vi "File.Remove Double Backslash from Path.vi"(11 "Path":path) -> (3 "Path Out":path)   [LabVIEW 2018]
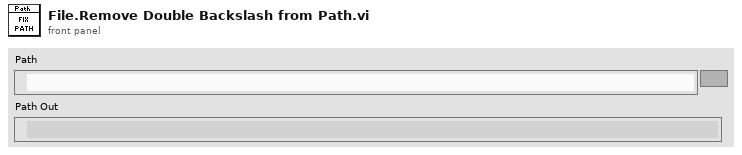
[diagram p1: front panel]
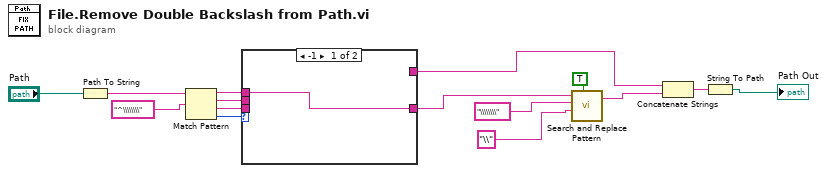
[diagram p0: block diagram]
diagram:
  n1 = Path To String(path="Path") -> (string=w14:string)
  n2 = Match Pattern(string=w14, regular expression="^\\\\\\\\") -> (before substring=w10:string, match substring=w9:string, after substring=w11:string, offset past match=w12:i32)  [unwired: 1 in]
  n3 = case shown="-1" w12 {
    tunnel: w11 -> [_ w18]
    tunnel: w10 -> [w16 _]
    tunnel: w9 -> [_ w17]
    tunnel: [w16 w18] -> w6
    tunnel: [_ w17] -> w3
    frame -1 {
    }
    frame 0, Default {
    }
  }
  n4 = call <vilib>:"Search and Replace Pattern.vi"("string"=w6, "regular expression (\"\")"="\\\\\\\\", "replace string (\"\")"="\\", "replace all? (F)"=TRUE) -> ("result string"=w4:string)  [unwired: 1 in, 1 out]
  n5 = Concatenate Strings(w3, w4) -> (w2:string)
  n6 = String To Path(string=w2) -> (path=→"Path Out":path)
